vi "GageLv_Core.vi"(8 "error in":errorcluster, 9 "SignalBuffer queue in":refnum<queue>, 10 "Gage CtrlQueue in":refnum<queue>) -> (0 "error out":errorcluster)   [LabVIEW 2014, in "GageLv.lvlib"]
uses:
  <instrlib>/GageLv_uic/GageLv.lvlib
  <instrlib>/GenericDAQ/VI/GenericDAQ_Ctrl_Queue.ctl
  <instrlib>/GenericDAQ/VI/GenericDAQ_State.ctl
  <instrlib>/GenericDAQ/VI/GenericDAQ_Signal.ctl
  <instrlib>/GageLv_uic/VI/Gage_Configs.ctl
  <instrlib>/GageLv_uic/VI/Gage_PrivateStats.ctl
  <instrlib>/GageLv_uic/VI/Gage_DAQStatus.ctl
  <vilib>/Utility/error.llb/DialogType.ctl
  <instrlib>/GageLv_uic/VI/SetSecondaryDataVIRef_Typedef.ctl
  <vilib>/Utility/error.llb/Error Cluster From Error Code.vi
  <vilib>/ErrorRing/Error Ring.xnode
  <userlib>/Utility/ErrorLog_lib.lvlib
  <instrlib>/GenericDAQ/GenericDAQ.lvlib
panel:
  in  "StartAll":bool
  out "Core#":i32
  in  "Get_ConfigAll":bool
  out "LiveStat":T1
  in  "Gage_Config":T3={"Acquisition"={"Sample Rate"=1000000000.0, "Mode"=0, "Start (0)"=0.0, "Depth"=32768.0, "Segment Size"=32768.0, "Trigger Delay"=0.0, "Trigger Timeout"=-1.0, "Trigger Holdoff"=0.0, "Clock mode"=enum."Internal", "Segment"=1}, "Channels"=[{"Coupling"=1, "Differential Input"=FALSE, "Direct-to-ADC"=FALSE, "Range"=2000, "Impedance"=50, "DC Offset"=0, "Filter"=0}], "Trigger"={"Slope"=0, "Level"=25, "Source"=0, "External Range"=2000, "External Coupling"=0, "External"=TRUE, "Disable"=FALSE, "External Impedance"=0}, "Mode(Gage)"=enum."Continuous"} {"Trigger"."External Impedance" items=["50 Ohm", "HiZ"]; "Trigger"."External Coupling" items=["DC", "AC"]; "Trigger"."External Range" min=2000 max=10000 step=8000; "Trigger"."Slope" items=["Rising", "Falling"]; "Trigger"."Level" min=-100 max=100; "Trigger"."Source" min=0 max=64 step=1; "Channels"."Impedance" min=50 max=1000000 step=999950; "Channels"."Coupling" items=["DC", "AC"]; "Acquisition"."Start (0)" min=-1000000.0 max=0.0 step=16.0; "Acquisition"."Segment Size" min=256.0 step=128.0; "Acquisition"."Trigger Delay" min=0.0 step=128.0; "Acquisition"."Trigger Timeout" format="%.0p"; "Acquisition"."Trigger Holdoff" min=0.0 step=128.0; "Acquisition"."Depth" min=256.0 step=128.0; "Acquisition"."Mode" items=["Single", "Dual", "Quad", "Octal"]; "Acquisition"."Sample Rate" format="%.0p"}
  out "Graph":sgl[](graph)
  in  "fConfig":bool
  in  "Reset":bool
  in  "CloseAll":bool
  in  "Close":bool
  in  "Enumerate":bool
  in  "Open":bool
  in  "Quit":bool
  in  "Start":bool
  in  "ConfigAll":bool
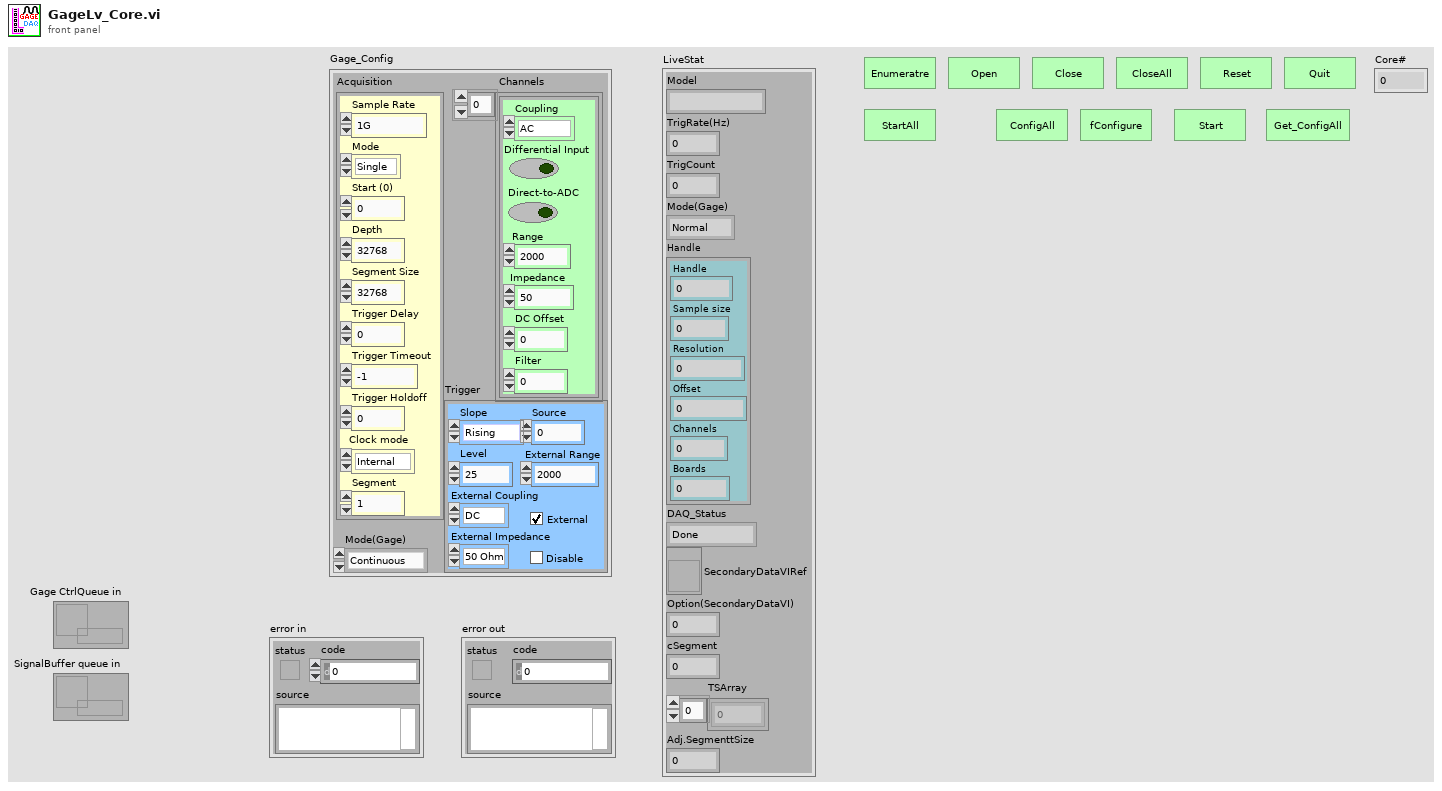
[diagram p1: front panel]
types:
  T1 = typedef "GageLv.lvlib/Gage_PrivateStats.ctl" = cluster{"Model":string, "TrigRate(Hz)":dbl, "TrigCount":i32, "Mode(Gage)":enum16{"Normal", "Continuous", "MultiRecord", "HwAverage"}, "Handle":cluster{"Handle":u32, "Sample size":u32, "Resolution":i32, "Offset":i32, "Channels":u32, "Boards":u32}, "DAQ_Status":T2, "SecondaryDataVIRef":refnum<vi>, "Option(SecondaryDataVI)":i32, "cSegment":i32, "TSArray":dbl[], "Adj.SegmenttSize":dbl}
  T2 = typedef "GageLv.lvlib/Gage_DAQStatus.ctl" = enum16{"Done", "Armed", "Triggered", "Transfering"}
  T3 = typedef "GageLv.lvlib/Gage_Configs.ctl" = cluster{"Acquisition":cluster{"Sample Rate":dbl, "Mode":u16, "Start (0)":dbl, "Depth":dbl, "Segment Size":dbl, "Trigger Delay":dbl, "Trigger Timeout":dbl, "Trigger Holdoff":dbl, "Clock mode":enum16{"Internal", "External", "Reference"}, "Segment":u32}, "Channels":cluster{"Coupling":u16, "Differential Input":bool, "Direct-to-ADC":bool, "Range":u32, "Impedance":u32, "DC Offset":i32, "Filter":i32}[], "Trigger":cluster{"Slope":u16, "Level":i32, "Source":i32, "External Range":u32, "External Coupling":u16, "External":bool, "Disable":bool, "External Impedance":u16}, "Mode(Gage)":enum16{"Normal", "Continuous", "MultiRecord", "HwAverage"}}
  T4 = enum16{"Normal", "MultiRecStart", "MultiRecEnd", "Reserved1", "Reserved2", "Reserved3"}
  T5 = typedef "DialogType.ctl" = u16
  T6 = typedef "GenericDAQ.lvlib/GenericDAQ_Signal.ctl" = cluster{"tickcount":u32, "Signal":sgl[], "SecondaryData":dbl[], "Flag":enum16{"Normal", "LineStart", "LineEnd", "FrameStart", "FrameEnd", "Reserved1", "Reserved2"}, "Segment#":i32}
  T7 = enum16{"Normal", "Continuous", "MultiRecord", "HwAverage"}
  T8 = typedef "GenericDAQ.lvlib/GenericDAQ_Ctrl_Queue.ctl" = cluster{"GenericDAQ State":T9, "Variant":variant}
  T9 = typedef "GenericDAQ.lvlib/GenericDAQ_State.ctl" = enum16{"Enumerate", "Open", "Close", "CloseAll", "Reset", "Quit", "==Settings==", "SetAcquisition_", "SetChannels_", "SetTrigger_", "SetAnalogTrigDetector_", "SetAll_AcquChTrig_", "fConfigurate", "fStart", "GetStatus", "_WaitForDone/Idle", "_GetData", "GetAcquisition", "GetChannels", "GetTrigger", "GetAll_AcquChTrig", "Abort", "==Messaging==", "_PushDataOut", "GetStat_", "GetConfig_", "==ModeSetup==", "SetSignalBuffer_", "SetMode_", "SetSecondaryDataRef._", "SetDynamicBuffer_", "==AnalogOut==", "GetChannelCount_AO", "fStart_AO", "SetChEnable_AO", "SetConfig_AO", "SetFuncData_AO", "SetOffset_AO_", "SetMasterNode_AO", "SetStates_AO", "SetSymetry_AO", "SetTriggerSource_AO", "==Trigger==", "ManualTrigger", "===Sync===", "LineStart", "LineEnd", "FrameStart", "FrameEnd", "EOL_PassThrough", "SOL_PassThrough"}
  T10 = typedef "SetSecondaryDataVIRef_Typedef.ctl" = cluster{"SecondaryDataVIRef.":refnum<vi>, "Option":i32}
  T11 = cluster{"Handle":u32, "Sample size":u32, "Resolution":i32, "Offset":i32, "Channels":u32, "Boards":u32}
  T12 = cluster{"Sample Rate":dbl, "Mode":u16, "Start (0)":dbl, "Depth":dbl, "Segment Size":dbl, "Trigger Delay":dbl, "Trigger Timeout":dbl, "Trigger Holdoff":dbl, "Clock mode":enum16{"Internal", "External", "Reference"}, "Segment":u32}
  T13 = cluster{"Sample Rate":dbl, "Clock mode":enum16{"Internal", "External", "Reference"}, string, "Depth":dbl, "Segment Size":dbl, "Trigger Timeout":dbl, "Trigger Holdoff":dbl, "Trigger Delay":dbl}
  T14 = cluster{"Coupling":u16, "Differential Input":bool, "Direct-to-ADC":bool, "Range":u32, "Impedance":u32, "DC Offset":i32, "Filter":i32}[]
  T15 = cluster{string, "Differential Input":bool, "Direct-to-ADC":bool, "Range":u32, "Impedance":u32, "DC Offset":i32, "Filter":i32}
  T16 = cluster{"Slope":u16, "Level":i32, "Source":i32, "External Range":u32, "External Coupling":u16, "External":bool, "Disable":bool, "External Impedance":u16}
  T17 = cluster{string, "Level":i32, "Source":i32, "External Range":u32, string, "External":bool, "Disable":bool, string}
  T18 = cluster{string, "Level":i32, "Source":i32, "External Range":u32, string, "External":bool, "Disable":bool, string}[]
  T19 = cluster{"Handle":u32, "Sample Size":u32, "Resolution":i32, "Offset":i32, "Channels":u32, "Boards":u32}
  T20 = cluster{"Coupling":u16, "Differential Input":bool, "Direct-to-ADC":bool, "Range":u32, "Impedance":u32, "DC Offset":i32, "Filter":i32}
  T21 = typedef "Gage.lvlib/Gage_Configs.ctl" = cluster{"Acquisition":cluster{"Sample Rate":dbl, "Mode":u16, "Start (0)":dbl, "Depth":dbl, "Segment Size":dbl, "Trigger Delay":dbl, "Trigger Timeout":dbl, "Trigger Holdoff":dbl, "Clock mode":enum16{"Internal", "External", "Reference"}, "Segment":u32}, "Channels":cluster{"Coupling":u16, "Differential Input":bool, "Direct-to-ADC":bool, "Range":u32, "Impedance":u32, "DC Offset":i32, "Filter":i32}[], "Trigger":cluster{"Slope":u16, "Level":i32, "Source":i32, "External Range":u32, "External Coupling":u16, "External":bool, "Disable":bool, "External Impedance":u16}, "Mode(Gage)":enum16{"Normal", "Continuous", "MultiRecord", "HwAverage"}}
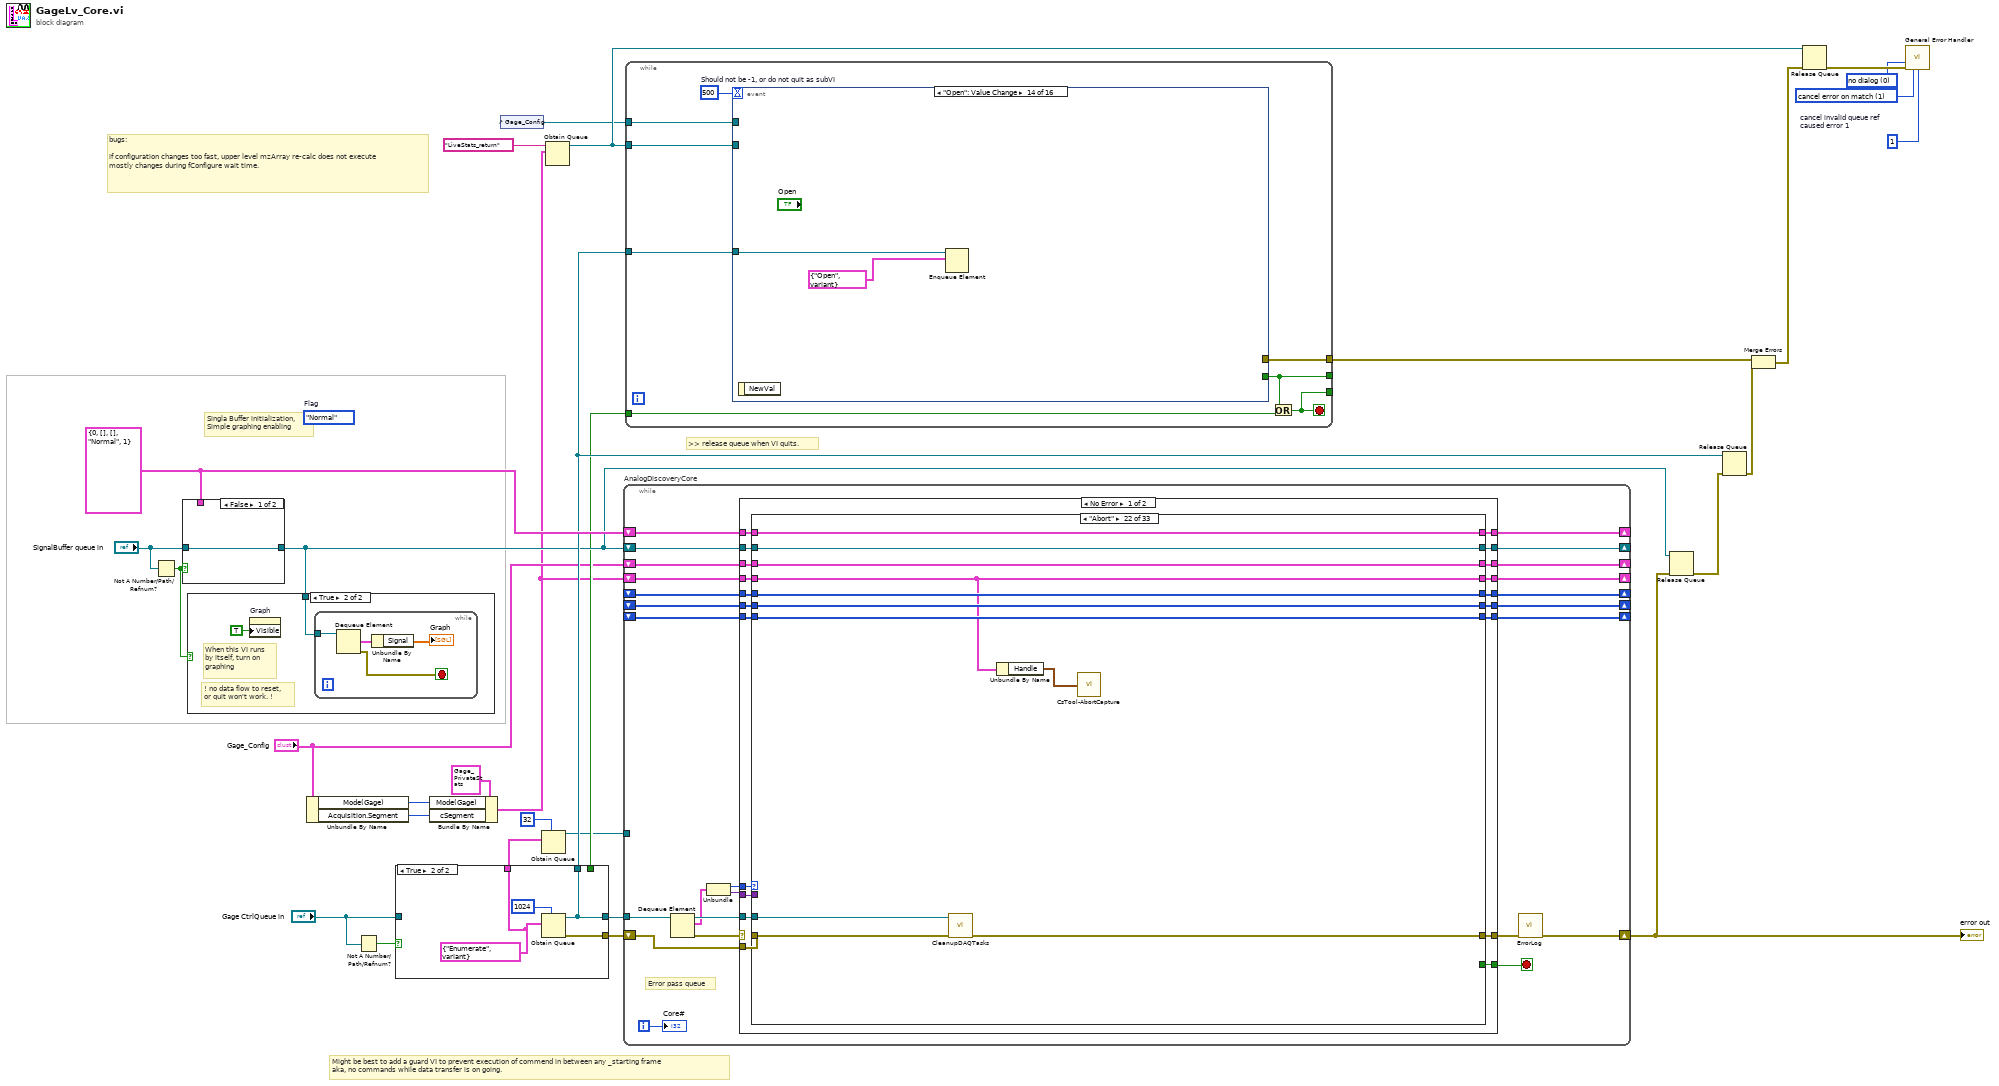
[diagram p0: block diagram]
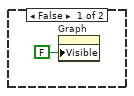
[diagram p2: hidden frame]
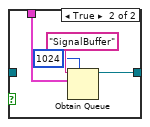
[diagram p3: hidden frame]
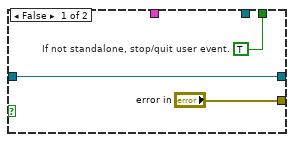
[diagram p4: hidden frame]
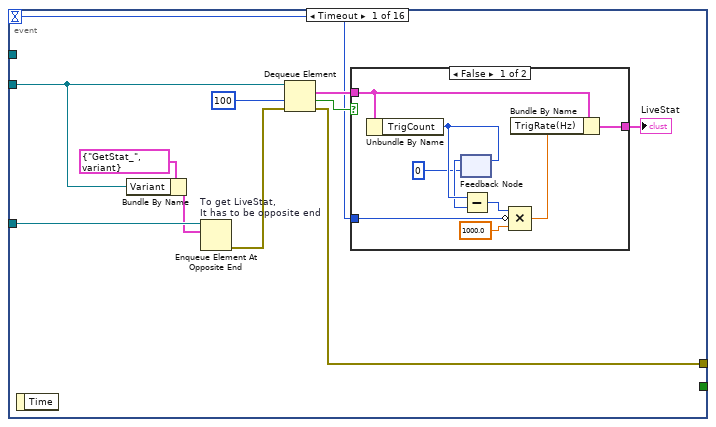
[diagram p5: hidden frame]
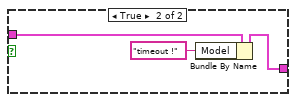
[diagram p6: hidden frame]
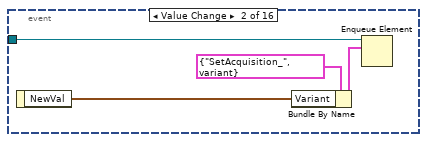
[diagram p7: hidden frame]
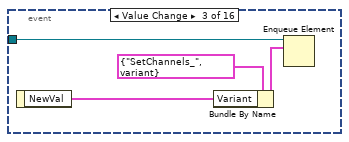
[diagram p8: hidden frame]
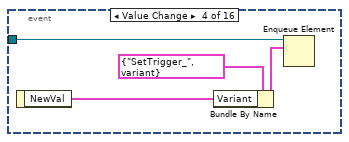
[diagram p9: hidden frame]
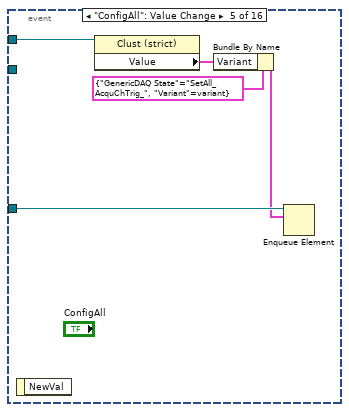
[diagram p10: hidden frame]
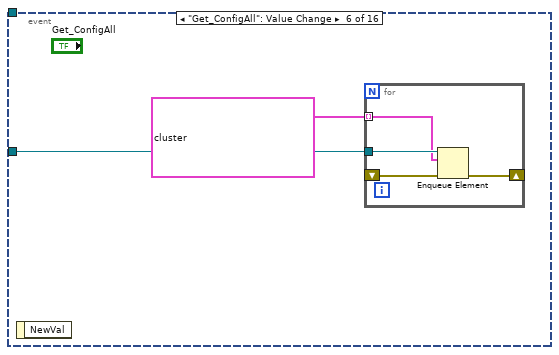
[diagram p11: hidden frame]
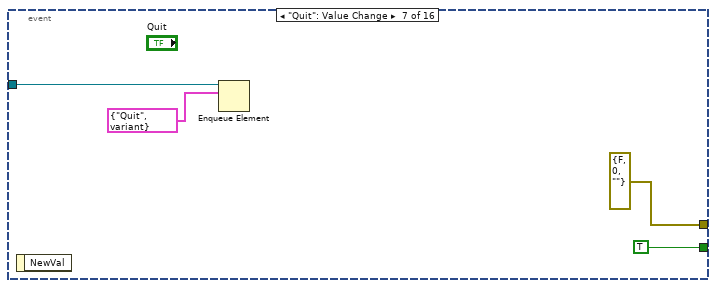
[diagram p12: hidden frame]
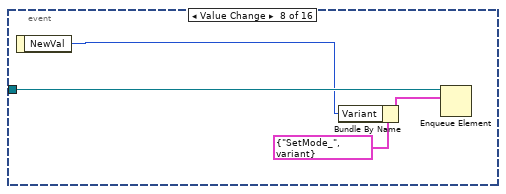
[diagram p13: hidden frame]
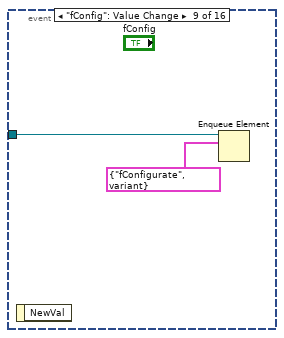
[diagram p14: hidden frame]
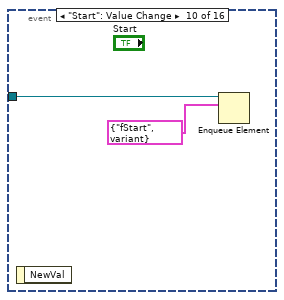
[diagram p15: hidden frame]
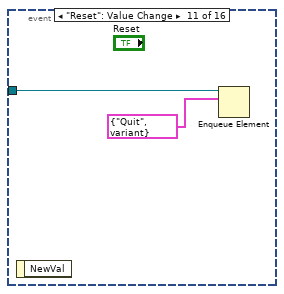
[diagram p16: hidden frame]
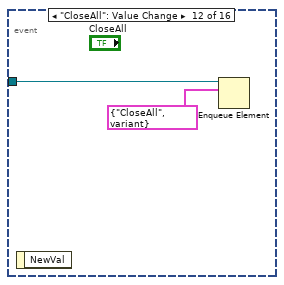
[diagram p17: hidden frame]
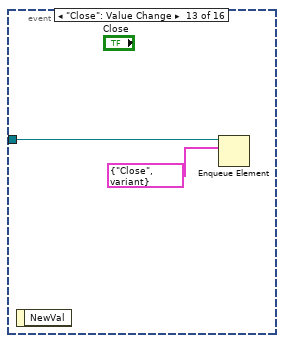
[diagram p18: hidden frame]
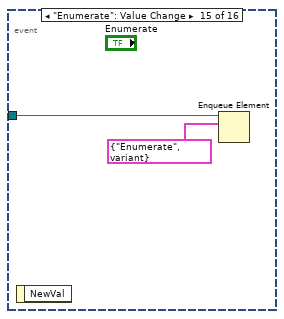
[diagram p19: hidden frame]
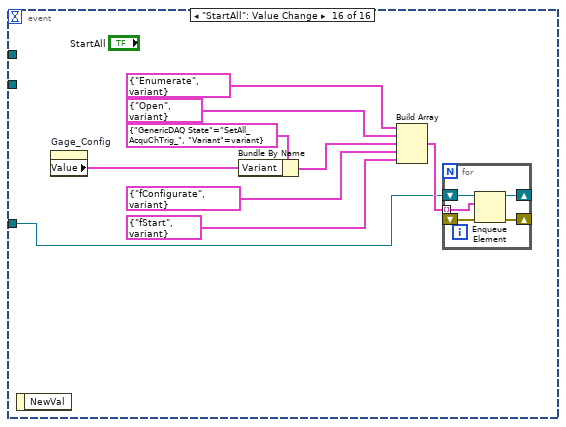
[diagram p20: hidden frame]
diagram:
  (unwired) T4."Normal"  # Flag
  w12 = 1  # cancel invalid queue ref caused error 1
  w13 = 1 items=["no exception", "cancel error on match", "set error on match"] ("[exception action] (none:0)")
  w14 = T5 0 items=["no dialog", "OK message", "continue or stop message", "OK message + warnings", "continue/stop + warnings"] ("type of dialog (OK msg:1)")
  w30 = T6 {"tickcount"=0, "Signal"=[], "SecondaryData"=[], "Flag"=enum."Normal", "Segment#"=1} ("Signal_Typedef")
  # "Might be best to add a guard VI to prevent execution of commend in between any _starting frame \naka, no commands while data transfer is on going."
  # "bugs:\n\nif configuration changes too fast, upper level mzArray re-calc does not execute\nmostly changes during fConfigure wait time."
  # "Singla Buffer initialization,\nSimple graphing enabling"
  # ">> release queue when VI quits."
  n1 = Not A Number/Path/Refnum?(number/path/refnum="SignalBuffer queue in") -> (NaN/Path/Refnum?=w17:bool)
  n2 = case shown="False" w17 {
    tunnel: w30 -> [_ w35]
    tunnel: [w31 w32] -> w18
    tunnel: "SignalBuffer queue in" -> [w31 _]
    frame False {
    }
    frame True {
      n3 = Obtain Queue(max queue size (-1, unlimited)=1024, name (unnamed)="SignalBuffer", element data type=w35) -> (queue out=w32:refnum<queue>)  [unwired: 2 in, 2 out]
    }
  }
  n4 = case shown="True" w17 {
    tunnel: w18 -> [_ w38]
    frame False {
      n5 = property on="Graph" class="WFGraph (strict)"("Visible"=FALSE) -> ()  [unwired: 2 in, 2 out]
    }
    frame True {
      # "! no data flow to reset,\nor quit won't work. !"
      # "When this VI runs\nby itself, turn on \ngraphing"
      n6 = property on="Graph" class="WFGraph (strict)"("Visible"=TRUE) -> ()  [unwired: 2 in, 2 out]
      n7 = while {
        tunnel: w38 -> [w42]
        stop <- w39 stop-if-true
        n8 = Dequeue Element(queue=w42) -> (element=w41:T6, error out=w39:errorcluster)  [unwired: 2 in, 2 out]
        n9 = Unbundle By Name(w41) -> ("Signal"=→"Graph":sgl[])
      }
    }
  }
  n10 = Unbundle By Name("Gage_Config") -> ("Mode(Gage)"=w8:T7, "Acquisition.Segment"=w1:u32)
  n11 = Not A Number/Path/Refnum?(number/path/refnum="Gage CtrlQueue in") -> (NaN/Path/Refnum?=w27:bool)
  n12 = case shown="True" w27 {
    tunnel: [w45 w47] -> w29
    tunnel: ["error in" w49] -> w28
    tunnel: "Gage CtrlQueue in" -> [w45 _]
    tunnel: [_ w47] -> w23
    tunnel: [w43 _] -> w11
    tunnel: [_ w46] -> w4
    frame False {
      w43 = TRUE  # If not standalone, stop/quit user event.
    }
    frame True {
      w46 = T8 {"GenericDAQ State"=enum."Enumerate", "Variant"=variant}
      n13 = Obtain Queue(max queue size (-1, unlimited)=1024, element data type=w46) -> (queue out=w47:refnum<queue>, error out=w49:errorcluster)  [unwired: 3 in, 1 out]
    }
  }
  n14 = Bundle By Name(cluster=T1 {"Model"="", "TrigRate(Hz)"=0.0, "TrigCount"=0, "Mode(Gage)"=enum."Normal", "Handle"={"Handle"=0, "Sample size"=0, "Resolution"=0, "Offset"=0, "Channels"=0, "Boards"=0}, "DAQ_Status"=enum."Done", "SecondaryDataVIRef"=refnum, "Option(SecondaryDataVI)"=0, "cSegment"=0, "TSArray"=[], "Adj.SegmenttSize"=0.0} ("PrivateStats(Live)"), "Mode(Gage)"=w8, "cSegment"=w1) -> (w5:T1)
  n15 = control-ref of="Gage_Config"() -> (w6:refnum<vi>)
  n16 = Obtain Queue(max queue size (-1, unlimited)=32, element data type=w4) -> (queue out=w3:refnum<queue>)  [unwired: 3 in, 2 out]
  n17 = Obtain Queue(name (unnamed)="LiveStats_return", element data type=w5) -> (queue out=w21:refnum<queue>)  [unwired: 3 in, 2 out]
  n18 = while "AnalogDiscoveryCore" {
    shift-right: [w73] -> _
    shift-left: w18 -> [w74]
    tunnel: w29 -> [w60]
    shift-right: [w50] -> w16
    shift-left: w28 -> [w62]
    shift-right: [w71] -> _
    shift-left: "Gage_Config" -> [w70]
    shift-right: [w54] -> _
    shift-left: w5 -> [w69]
    shift-right: [w63] -> _
    shift-left: _ -> [w67]
    shift-right: [w64] -> _
    shift-left: w30 -> [w68]
    shift-right: [w57] -> _
    shift-left: _ -> [w55]
    shift-right: [w58] -> _
    shift-left: _ -> [w56]
    tunnel: w3 -> [_]
    i -> [w52]
    stop <- w72 stop-if-true
    # "Error pass queue"
    n19 = Dequeue Element(queue=w60) -> (queue out=w59:refnum<queue>, element=w53:T8, error out=w61:errorcluster)  [unwired: 2 in, 1 out]
    n20 = Unbundle(w53) -> ("GenericDAQ State"=w66:T9, "Variant"=w65:variant)
    n21 = case shown="No Error" w61 {
      tunnel: w74 -> [w94 w1020]
      tunnel: [w93 w1020] -> w73
      tunnel: [w92 TRUE] -> w72
      tunnel: [w91 w1018] -> w51
      tunnel: [w90 w1021] -> w71
      tunnel: w70 -> [w89 w1021]
      tunnel: w69 -> [w88 w1022]
      tunnel: w68 -> [w87 w1019]
      tunnel: w67 -> [w86 w1023]
      tunnel: w59 -> [w85 _]
      tunnel: w66 -> [w84 _]
      tunnel: w65 -> [w83 _]
      tunnel: [w82 w1019] -> w64
      tunnel: [w81 w1023] -> w63
      tunnel: [w80 w1022] -> w54
      tunnel: w62 -> [w79 _]
      tunnel: [w78 w1017] -> w58
      tunnel: [w77 w1016] -> w57
      tunnel: w56 -> [w76 w1017]
      tunnel: w55 -> [w75 w1016]
      frame No Error {
        n22 = case shown="\"Abort\"" w84 {
          tunnel: w94 -> [w102 w111 w140 w153 w169 w184 w201 w219 w242 w313 w368 w423 w468 w491 w507 w529 w585 w675 w690 w733 w744 w759 w767 w800 w887 w900 w913 w926 w952 w966 w997 w998 w1007]
          tunnel: [w102 w111 w140 w153 w169 w184 w201 w219 w242 w313 w368 w423 w468 w491 w507 w529 w585 w675 w690 w733 w744 w759 w767 w800 w887 w900 w913 w927 w952 w966 w997 w998 w1007] -> w93
          tunnel: [_ _ _ _ _ _ w195 _ _ _ _ _ _ _ _ _ _ _ _ _ _ _ _ _ _ _ _ _ _ _ _ _ _] -> w92
          tunnel: w85 -> [_ _ _ _ _ w180 w192 _ w225 w299 w354 w420 w455 w485 _ w531 w581 _ _ _ w737 w751 _ w796 _ _ _ _ _ _ _ _ _]
          tunnel: w79 -> [w101 w107 w136 w147 w168 w179 w193 _ w234 w304 w359 w414 w456 w475 w503 w530 w579 w674 w689 w732 w736 w750 _ w798 w881 w891 _ w923 w942 _ w996 w1006 w1015]
          tunnel: [w101 w107 errorcluster {"status"=FALSE, "code"=0, "source"=""} ("error out") w142 w161 w178 w194 w214 w230 w305 w360 w419 w453 w479 w503 w524 w582 w652 w678 w707 w735 w749 w762 w797 w880 w892 w908 w924 w943 w954 w996 w1006 w1015] -> w91
          tunnel: [w100 w110 w139 w152 w167 w183 w200 w218 w239 w310 w365 w417 w467 w490 w506 w528 w587 w669 w685 w725 w740 w758 w766 w791 w879 w893 w912 w932 w951 w965 w995 w1005 w1014] -> w90
          tunnel: w89 -> [w100 w110 w139 w152 w167 w183 w200 w218 w237 w308 w363 w417 w467 w490 w506 w528 w587 w671 w683 w731 w740 w758 w766 w791 w879 w893 w912 w932 w951 w965 w995 w1005 w1014]
          tunnel: [w99 w109 w131 w149 w162 w177 w197 w217 w240 w311 w366 w411 w465 w488 w502 w521 w554 w665 w684 w726 w743 w752 w765 w781 w876 w899 w911 w931 w948 w960 w994 w1004 w1013] -> w80
          tunnel: w88 -> [w99 w109 w137 w150 w162 w177 w197 w217 w240 w311 w366 w411 w465 w488 w498 w522 w576 w670 w684 w726 w743 w752 w765 w782 w876 w899 w911 w931 w947 w955 w994 w1004 w1013]
          tunnel: w87 -> [w98 w108 w138 w151 w166 w182 w199 w216 w241 w312 w367 w422 w466 w489 w505 w527 w584 w673 w688 w730 w742 w757 w764 w775 w886 w898 w910 w930 w950 w964 w993 w1003 w1012]
          tunnel: w86 -> [w97 w106 _ w148 w165 w181 w198 w215 w231 w302 w357 w421 w464 w484 w504 w523 w586 w672 w687 w729 w741 w756 w763 w789 w885 w897 w909 w929 w949 w963 w992 w1002 w1011]
          tunnel: w83 -> [_ _ w135 _ _ _ _ _ w238 w309 w364 w418 _ _ _ _ _ _ _ _ _ _ _ _ w882 w896 _ w928 w946 w958 _ _ _]
          tunnel: [w98 w108 w138 w151 w166 w182 w199 w216 w241 w312 w367 w422 w466 w489 w505 w527 w583 w673 w688 w730 w742 w757 w764 w775 w886 w898 w910 w930 w950 w964 w993 w1003 w1012] -> w82
          tunnel: [w97 w106 w115 w148 w165 w181 w198 w215 w232 w302 w357 w421 w464 w484 w504 w523 w578 w672 w687 w729 w741 w756 w763 w788 w885 w897 w909 w929 w949 w963 w992 w1002 w1011] -> w81
          tunnel: [w96 w104 w114 w146 w164 w171 w191 w213 w229 w301 w356 w413 w462 w483 w501 w511 w570 w659 w680 w728 w739 w755 w761 w786 w878 w890 w907 w920 w941 w962 w991 w1001 w1010] -> w78
          tunnel: [w95 w103 w113 w145 w163 w170 w190 w212 w228 w300 w355 w412 w461 w482 w500 w510 w569 w658 w679 w727 w738 w754 w760 w784 w877 w889 w906 w919 w940 w961 w990 w1000 w1009] -> w77
          tunnel: w76 -> [w96 w104 _ w146 w164 w171 w191 w213 w227 w301 w356 w413 w462 w483 w501 w511 w573 w659 w680 w728 w739 w755 w761 w787 w878 w890 w907 w920 w941 w962 w991 w1001 w1010]
          tunnel: w75 -> [w95 w103 _ w145 w163 w170 w190 w212 w226 w300 w355 w412 w461 w482 w500 w510 w572 w658 w679 w727 w738 w754 w760 w785 w877 w889 w906 w919 w940 w961 w990 w1000 w1009]
          frame Default {
          }
          frame "Enumerate" {
            n23 = call <instrlib>:"CsTool-Initialize.vi"() -> ("Number Of Systems"=w105:i32)  [unwired: 1 out]
            n24 = call <instrlib>:"CsTool-ErrorHandler.vi"("Error Code"=w105) -> ()  [unwired: 2 in, 1 out]
          }
          frame "Open" {
            n25 = Variant To Data(error in=w136, type="", Variant=w135) -> (data=w130:string, error out=w133:errorcluster)
            n26 = Select(t="any", s=TRUE, f=w130) -> (s? t:f=w129:string)
            n27 = call <instrlib>:"CsTool-GetSystem.vi"("Board Name (Any)"=w129) -> ("Error Code"=w132:i32, "Handle Cluster"=w121:T11)  [unwired: 3 in]
            n28 = call <instrlib>:"CsTool-GetSystemName.vi"("Handle Cluster"=w121) -> ()  [unwired: 2 out]
            n29 = call <instrlib>:"CsTool-ErrorHandler.vi"("Error Code"=w132, "Handle Cluster"=w121) -> ("Error String"=w122:string)  [unwired: 1 in]
            n30 = call <instrlib>:"CsTool-GetSystemInfo.vi"("Handle Cluster"=w121) -> ()  [unwired: 7 out]
            n31 = Bundle By Name(cluster=w137, "Handle"=w121, "Model"=w129, "TrigRate(Hz)"=0.0, "TrigCount"=0) -> (w131:T1)
            n32 = Bundle By Name(cluster=w133, "source"=w122) -> ()  [unwired: 1 out]
            n33 = Wait (ms)(milliseconds to wait=u32 0) -> ()  [unwired: 1 out]
            n34 = Multiply(x=2 ("16KSa, per spec"), y=262144 ("dimension size")) -> (x*y=w116:i32)
            n35 = Initialize Array(0 ("Numeric"), w116) -> (w115:i32[])
            n36 = Initialize Array(i16 0 ("Numeric"), w116) -> (w114:i16[])
            n37 = Initialize Array(u8 0 ("Numeric"), w116) -> (w113:u8[])
          }
          frame "Close" {
            n38 = Unbundle By Name(w150) -> ("Handle"=w143:T11)
            n39 = call <instrlib>:"CsTool-AbortCapture.vi"("Handle Cluster"=w143) -> ("Error Code"=w144:i32)
            n40 = call <instrlib>:"CsTool-ErrorHandler.vi"("Error Code"=w144, "Handle Cluster"=w143) -> ("Error String"=w141:string)  [unwired: 1 in]
            n41 = disable-structure shown="Enabled" {
              disable-tunnel: w150 -> [w156 w157]
              disable-tunnel: [w155 w157] -> w149
              frame Enabled {
                n42 = Bundle By Name(cluster=w156, "Handle.Handle"=u32 0) -> (w155:T1)
              }
              frame Disabled {
              }
            }
            n43 = Bundle By Name(cluster=w147, "source"=w141) -> (w142:errorcluster)
          }
          frame "CloseAll" {
            # "not really useful here."
            n44 = Unbundle By Name(w162) -> ("Handle"=w160:T11)
            n45 = call <instrlib>:"CsTool-AbortCapture.vi"("Handle Cluster"=w160) -> ("Error Code"=w159:i32)
            n46 = call <instrlib>:"CsTool-ErrorHandler.vi"("Error Code"=w159, "Handle Cluster"=w160) -> ("Error String"=w158:string)  [unwired: 1 in]
            n47 = Bundle By Name(cluster=w168, "source"=w158) -> (w161:errorcluster)
          }
          frame "Reset" {
            n48 = Unbundle By Name(w177) -> ("Model"=w175:string)
            n49 = Bundle By Name(cluster=T8 {"GenericDAQ State"=enum."Open", "Variant"=variant} ("element"), "Variant"=w175) -> (w174:T8)
            n50 = Build Array(w174, T8 {"GenericDAQ State"=enum."Close", "Variant"=variant} ("element")) -> (w172:T8[])
            n51 = for {
              tunnel: w180 -> [w188]
              tunnel: w172 -> [w185] mode=indexing
              shift-right: [w186] -> w178
              shift-left: w179 -> [w187]
              n52 = Enqueue Element At Opposite End(queue=w188, element=w185, error in (no error)=w187) -> (error out=w186:errorcluster)  [unwired: 1 in, 2 out]
            }
          }
          frame "Quit" {
            n53 = Unbundle By Name(w197) -> ("Handle"=w189:T11, "Handle.Handle"=w196:u32)
            n54 = case "Check handle leak??" shown="Default" w196 {
              tunnel: [_ TRUE] -> w195
              tunnel: [w203 _] -> w194
              tunnel: w193 -> [w204 _]
              tunnel: w192 -> [w205 _]
              tunnel: w189 -> [_ w210]
              frame Default {
                n55 = for {
                  tunnel: w205 -> [w209]
                  tunnel: T8[] [{"GenericDAQ State"=enum."Quit", "Variant"=variant}, {"GenericDAQ State"=enum."Close", "Variant"=variant}] -> [w206] mode=indexing
                  shift-right: [w207] -> w203
                  shift-left: w204 -> [w208]
                  n56 = Enqueue Element At Opposite End(queue=w209, element=w206, error in (no error)=w208) -> (error out=w207:errorcluster)  [unwired: 1 in, 2 out]
                }
              }
              frame 0 {
                n57 = call <instrlib>:"CsTool-FreeSystem.vi"("Handle Cluster"=w210) -> ()  [unwired: 1 out]
              }
            }
          }
          frame "==Settings==" {
            # "Invalid frame"
            n58 = xnode "Error Ring"() -> ("error out"=w214:errorcluster)
          }
          frame "SetAcquisition_" {
            n59 = Unbundle By Name(w237) -> ("Acquisition"=w236:T12)
            n60 = Variant To Data(error in=w234, type=w236, Variant=w238) -> (data=w235:T12, error out=w233:errorcluster)
            n61 = Bundle By Name(cluster=w237, "Acquisition"=w235) -> (w239:T3)
            n62 = case shown="No Error" w233 {
              selector: w233 -> [w250 _]
              tunnel: w240 -> [w277 _]
              tunnel: w235 -> [w270 _]
              tunnel: [w263 w293] -> w232
              tunnel: w231 -> [_ w293]
              tunnel: [w260 w292] -> w230
              tunnel: [w262 w291] -> w229
              tunnel: [w261 w290] -> w228
              tunnel: w227 -> [_ w291]
              tunnel: w226 -> [_ w290]
              tunnel: w225 -> [w251 _]
              frame No Error {
                n63 = call <instrlib>:"CleanupDAQTasks.vi"("error in (no error)"=w250, "Queue in"=w251) -> ("error out"=w249:errorcluster)  [unwired: 8 in, 1 out]
                n64 = Unbundle By Name(w270) -> ("Segment"=w246:u32, "Mode"=w257:u16, "Sample Rate"=w276:dbl, "Clock mode"=w275:enum16{"Internal", "External", "Reference"})
                n65 = Unbundle By Name(w270) -> ("Depth"=w267:dbl, "Segment Size"=w274:dbl, "Trigger Timeout"=w273:dbl, "Trigger Holdoff"=w272:dbl, "Trigger Delay"=w271:dbl)
                n66 = Unbundle By Name(w277) -> ("Handle"=w259:T11)
                n67 = flat-sequence {
                  tunnel: w259 -> [w281]
                  tunnel: [w281] -> _
                  tunnel: [w281] -> w247
                  tunnel: [w282] -> w248
                  tunnel: w247 -> [w282]
                  tunnel: w248 -> [w289]
                  tunnel: w246 -> [w288]
                  tunnel: w245 -> [w287]
                  tunnel: [w286] -> w244
                  tunnel: [w285] -> w243
                  frame #0 {
                    n68 = call <instrlib>:"CsTool-AbortCapture.vi"("Handle Cluster"=w281) -> ()  [unwired: 1 out]
                  }
                  frame #1 {
                    n69 = Wait (ms)(milliseconds to wait=u32 5) -> ()  [unwired: 1 out]
                  }
                  frame #2 {
                    n70 = call <instrlib>:"CsTool-ConfigureAcquisition.vi"("Handle Cluster"=w289, "Segment Count (1)"=w288, "Acquisition"=w287) -> ("Error Code"=w285:i32)  [unwired: 2 in]
                    n71 = call <instrlib>:"CsTool-ErrorHandler.vi"("StopOnError (true)"=FALSE, "Error Code"=w285, "Handle Cluster"=w289) -> ("Error String"=w286:string)
                  }
                }
                n72 = Index Array(array=string[] ["Single", "Dual", "Quad", "Octal"], index=w257) -> (element=w268:string)
                n73 = Scale By Power Of 2(n=w257, x=ext 1.0) -> (x*2^n=w258:ext)
                n74 = To Long Integer(number=w258) -> (32bit integer=w253:i32)
                n75 = Bundle("Sample Rate"=w276, "Clock mode"=w275, w268, "Depth"=w267, "Segment Size"=w274, "Trigger Timeout"=w273, "Trigger Holdoff"=w272, "Trigger Delay"=w271) -> (w245:T13)  [unwired: 1 in]
                n76 = Less Than 0?(x=w243) -> (x < 0?=w255:bool)
                n77 = To Long Integer(number=w267) -> (32bit integer=w266:i32)
                n78 = In Range and Coerce(upper limit=512000, x=w266, lower limit=1) -> (coerced(x)=w254:i32)  [unwired: 1 out]
                n79 = Multiply(x=w253, y=w254) -> (x*y=w252:i32)
                n80 = Initialize Array(0 ("Numeric"), w252) -> (w263:i32[])
                n81 = Initialize Array(i16 0 ("Numeric"), w252) -> (w262:i16[])
                n82 = Initialize Array(u8 0 ("Numeric"), w252) -> (w261:u8[])
                n83 = Bundle By Name(cluster=w249, "status"=w255, "source"=w244) -> (w260:errorcluster)
              }
              frame Error {
                n84 = xnode "Error Ring"() -> ("error out"=w292:errorcluster)
              }
            }
          }
          frame "SetChannels_" {
            n85 = Unbundle By Name(w308) -> ("Channels"=w307:T14)
            n86 = Variant To Data(error in=w304, type=w307, Variant=w309) -> (data=w306:T14, error out=w303:errorcluster)
            n87 = Bundle By Name(cluster=w308, "Channels"=w306) -> (w310:T3)
            n88 = case shown="No Error" w303 {
              selector: w303 -> [w324 _]
              tunnel: w311 -> [w327 _]
              tunnel: w306 -> [w326 _]
              tunnel: [w323 w348] -> w305
              tunnel: w299 -> [w320 _]
              frame No Error {
                n89 = call <instrlib>:"CleanupDAQTasks.vi"("error in (no error)"=w324, "Queue in"=w320) -> ("error out"=w321:errorcluster)  [unwired: 8 in, 1 out]
                n90 = for {
                  tunnel: w326 -> [w337] mode=indexing
                  shift-right: [w347] -> w325
                  shift-left: w321 -> [w347]
                  tunnel: [w336] -> w318 mode=indexing
                  n91 = Unbundle By Name(w337) -> ("Coupling"=w340:u16, "Differential Input"=w338:bool, "Direct-to-ADC"=w341:bool, "Range"=w342:u32, "Impedance"=w343:u32, "DC Offset"=w344:i32, "Filter"=w345:i32)
                  n92 = Index Array(array=string[] ["DC", "AC"] ("Strings []"), index=w340) -> (element=w339:string)
                  n93 = Bundle(w339, "Differential Input"=w338, "Direct-to-ADC"=w341, "Range"=w342, "Impedance"=w343, "DC Offset"=w344, "Filter"=w345) -> (w336:T15)  [unwired: 1 in]
                }
                n94 = Unbundle By Name(w327) -> ("Handle"=w322:T11)
                n95 = flat-sequence {
                  tunnel: w322 -> [w328]
                  tunnel: [w328] -> w317
                  tunnel: w317 -> [w330]
                  tunnel: [w330] -> w316
                  tunnel: w316 -> [w333]
                  tunnel: [w335] -> w319
                  tunnel: w318 -> [w334]
                  tunnel: [w331] -> w314
                  frame #0 {
                    n96 = call <instrlib>:"CsTool-AbortCapture.vi"("Handle Cluster"=w328) -> ()  [unwired: 1 out]
                  }
                  frame #1 {
                    n97 = Wait (ms)(milliseconds to wait=u32 5) -> ()  [unwired: 1 out]
                  }
                  frame #2 {
                    n98 = call <instrlib>:"CsTool-ConfigureChannelArray.vi"("Channels"=w334, "Handle Cluster"=w333) -> ("Error Code"=w331:u32)
                    n99 = call <instrlib>:"CsTool-ErrorHandler.vi"("StopOnError (true)"=FALSE, "Error Code"=w331, "Handle Cluster"=w333) -> ("Error String"=w335:string)
                  }
                }
                n100 = Less Than 0?(x=w314) -> (x < 0?=w315:bool)
                n101 = Bundle By Name(cluster=w325, "status"=w315, "source"=w319) -> (w323:errorcluster)
              }
              frame Error {
                n102 = xnode "Error Ring"() -> ("error out"=w348:errorcluster)
              }
            }
          }
          frame "SetTrigger_" {
            n103 = Unbundle By Name(w363) -> ("Trigger"=w362:T16)
            n104 = Variant To Data(error in=w359, type=w362, Variant=w364) -> (data=w361:T16, error out=w358:errorcluster)
            n105 = Bundle By Name(cluster=w363, "Trigger"=w361) -> (w365:T3)
            n106 = case shown="No Error" w358 {
              selector: w358 -> [w395 _]
              tunnel: w366 -> [w396 _]
              tunnel: w361 -> [w388 _]
              tunnel: [w378 w405] -> w360
              tunnel: w354 -> [w373 _]
              frame No Error {
                n107 = call <instrlib>:"CleanupDAQTasks.vi"("error in (no error)"=w395, "Queue in"=w373) -> ("error out"=w374:errorcluster)  [unwired: 8 in, 1 out]
                n108 = Unbundle By Name(w388) -> ("Slope"=w384:u16, "Level"=w391:i32, "Source"=w390:i32, "External Range"=w389:u32, "External Coupling"=w383:u16, "External"=w394:bool, "Disable"=w393:bool, "External Impedance"=w382:u16)
                n109 = Unbundle By Name(w396) -> ("Handle"=w377:T11)
                n110 = Index Array(array=string[] ["Rising", "Falling"] ("Strings [] 3"), index=w384) -> (element=w381:string)
                n111 = Index Array(array=string[] ["DC", "AC"] ("Strings [] 2"), index=w383) -> (element=w380:string)
                n112 = Index Array(array=string[] ["50 Ohm", "HiZ"] ("Strings []"), index=w382) -> (element=w379:string)
                n113 = flat-sequence {
                  tunnel: w377 -> [w397]
                  tunnel: [w397] -> w372
                  tunnel: w372 -> [w399]
                  tunnel: [w399] -> w371
                  tunnel: w371 -> [w402]
                  tunnel: w376 -> [w404]
                  tunnel: [w403] -> w375
                  tunnel: [w400] -> w369
                  frame #0 {
                    n114 = call <instrlib>:"CsTool-AbortCapture.vi"("Handle Cluster"=w397) -> ()  [unwired: 1 out]
                  }
                  frame #1 {
                    n115 = Wait (ms)(milliseconds to wait=u32 5) -> ()  [unwired: 1 out]
                  }
                  frame #2 {
                    n116 = call <instrlib>:"CsTool-ConfigureTriggerArray.vi"("Triggers"=w404, "Handle Cluster"=w402) -> ("Error Code"=w400:i32)
                    n117 = call <instrlib>:"CsTool-ErrorHandler.vi"("StopOnError (true)"=FALSE, "Error Code"=w400, "Handle Cluster"=w402) -> ("Error String"=w403:string)
                  }
                }
                n118 = Bundle(w381, "Level"=w391, "Source"=w390, "External Range"=w389, w380, "External"=w394, "Disable"=w393, w379) -> (w392:T17)  [unwired: 1 in]
                n119 = Build Array(w392) -> (w376:T18)
                n120 = Less Than 0?(x=w369) -> (x < 0?=w370:bool)
                n121 = Bundle By Name(cluster=w374, "status"=w370, "source"=w375) -> (w378:errorcluster)
              }
              frame Error {
                n122 = xnode "Error Ring"() -> ("error out"=w405:errorcluster)
              }
            }
          }
          frame "SetAll_AcquChTrig_" {
            n123 = Variant To Data(type=w417, Variant=w418) -> (data=w415:T3, error out=w416:errorcluster)  [unwired: 1 in]
            n124 = case shown="No Error" w416 {
              tunnel: w420 -> [w441 _]
              tunnel: [w440 w446] -> w419
              tunnel: w415 -> [w439 _]
              tunnel: w414 -> [w438 _]
              frame No Error {
                n125 = Unbundle By Name(w439) -> ("Mode(Gage)"=w428:T7, "Acquisition"=w436:T12, "Channels"=w434:T14, "Trigger"=w432:T16)
                n126 = Bundle By Name(cluster=T8 {"GenericDAQ State"=enum."SetMode_", "Variant"=variant} ("element"), "Variant"=w428) -> (w425:T8)
                n127 = Bundle By Name(cluster=T8 {"GenericDAQ State"=enum."SetAcquisition_", "Variant"=variant} ("element"), "Variant"=w436) -> (w426:T8)
                n128 = Bundle By Name(cluster=T8 {"GenericDAQ State"=enum."SetChannels_", "Variant"=variant} ("element"), "Variant"=w434) -> (w424:T8)
                n129 = Bundle By Name(cluster=T8 {"GenericDAQ State"=enum."SetTrigger_", "Variant"=variant} ("element"), "Variant"=w432) -> (w431:T8)
                n130 = Build Array(w425, w426, w424, w431) -> (w430:T8[])
                n131 = Reverse 1D Array(array=w430) -> (reversed array=w427:T8[])
                n132 = for "Has to be at the \nopposite end, otherwise\nrace condition" {
                  tunnel: w441 -> [w445]
                  shift-right: [w444] -> w440
                  shift-left: w438 -> [w443]
                  tunnel: w427 -> [w442] mode=indexing
                  n133 = Enqueue Element At Opposite End(queue=w445, element=w442, error in (no error)=w443) -> (error out=w444:errorcluster)  [unwired: 1 in, 2 out]
                }
              }
              frame Error {
                n134 = xnode "Error Ring"() -> ("error out"=w446:errorcluster)
              }
            }
          }
          frame "fConfigurate" {
            # "If dependancy of ErrorLog missing, \njust remove errorlog vi."
            # "fConfigurate => Commit (as in Gage SDK)"
            n135 = call <instrlib>:"CleanupDAQTasks.vi"("error in (no error)"=w456, "Queue in"=w455) -> ("error out"=w457:errorcluster)  [unwired: 8 in, 1 out]
            n136 = Unbundle By Name(w465) -> ("Handle"=w463:T11)
            n137 = flat-sequence {
              tunnel: w463 -> [w469]
              tunnel: [w469] -> w460
              tunnel: w460 -> [w472]
              tunnel: [w473] -> w458
              tunnel: [w471] -> w452
              frame #0 {
                n138 = disable-structure shown="Enabled" {
                  disable-tunnel: w469 -> [w470 _]
                  frame Enabled {
                    n139 = call <instrlib>:"CsTool-AbortCapture.vi"("Handle Cluster"=w470) -> ()  [unwired: 1 out]
                  }
                  frame Disabled {
                  }
                }
              }
              frame #1 {
                n140 = call <instrlib>:"CsTool-Commit.vi"("Handle Cluster"=w472) -> ("Error Code"=w471:i32)  [unwired: 2 in, 1 out]
                n141 = call <instrlib>:"CsTool-ErrorHandler.vi"("StopOnError (true)"=FALSE, "Error Code"=w471, "Handle Cluster"=w472) -> ("Error String"=w473:string)
              }
            }
            n142 = Less Than 0?(x=w452) -> (x < 0?=w454:bool)
            n143 = Bundle By Name(cluster=w457, "code"=w452, "status"=w454, "source"=w458) -> (w459:errorcluster)
            n144 = call <userlib>:"ErrorLog.vi"("error in (no error)"=w459) -> ("error out"=w453:errorcluster)  [unwired: 10 in]
          }
          frame "fStart" {
            # "Known issue:\n\nIf too manu fStart send here, virtual system crash.\nhas to restart Lv"
            # "Prevent program termination, \nwhen capture executed \nbefore previous one finished\n\nCould not find how to detect\na unfinished capture\n\nIn GetDate frame, capture actions is \nguarentted finished, no need to do so."
            n145 = call <instrlib>:"CleanupDAQTasks.vi"("error in (no error)"=w475, "Queue in"=w485) -> ("error out"=w476:errorcluster, "Queue out"=w477:refnum<queue>)  [unwired: 8 in]
            n146 = Unbundle By Name(w488) -> ("Handle"=w481:T11)
            n147 = flat-sequence {
              tunnel: w481 -> [w493]
              tunnel: [w493] -> w480
              tunnel: w480 -> [w495]
              tunnel: [w494] -> w478
              frame #0 {
                n148 = Wait (ms) "Prevent termination if too many \nfStart sent in short time."(milliseconds to wait=u32 50) -> ()  [unwired: 1 out]
                n149 = call <instrlib>:"CsTool-AbortCapture.vi"("Handle Cluster"=w493) -> ()  [unwired: 1 out]
              }
              frame #1 {
                n150 = call <instrlib>:"CsTool-Capture.vi"("Handle Cluster"=w495) -> ("Error Code"=w496:i32)
                n151 = call <instrlib>:"CsTool-ErrorHandler.vi"("Error Code"=w496, "Handle Cluster"=w495) -> ("Error String"=w494:string)  [unwired: 1 in]
              }
            }
            n152 = Enqueue Element(queue=w477, element=T8 {"GenericDAQ State"=enum."_WaitForDone/Idle", "Variant"=variant}, error in (no error)=w476) -> (error out=w486:errorcluster)  [unwired: 1 in, 2 out]
            n153 = Bundle By Name(cluster=w486, "source"=w478) -> (w479:errorcluster)
          }
          frame "GetStatus" {
            n154 = Unbundle By Name(w498) -> ("Handle"=w499:T11)
            n155 = call <instrlib>:"CsTool-QueryStatus.vi"("Handle Cluster"=w499) -> ("Status"=w497:i32)
            n156 = Bundle By Name(cluster=w498, "DAQ_Status"=w497) -> (w502:T1)
          }
          frame "_WaitForDone/Idle" {
            w517 = T9[] [enum."Close", enum."CloseAll", enum."Reset", enum."Quit", enum."Abort"] items=["Enumerate", "Open", "Close", "CloseAll", "Reset", "Quit", "==Settings==", "SetAcquisition_", "SetChannels_", "SetTrigger_", "SetAnalogTrigDetector_", "SetAll_AcquChTrig_", "fConfigurate", "fStart", "GetStatus", "_WaitForDone/Idle", "_GetData", "GetAcquisition", "GetChannels", "GetTrigger", "GetAll_AcquChTrig", "Abort", "==Messaging==", "_PushDataOut", "GetStat_", "GetConfig_", "==ModeSetup==", "SetSignalBuffer_", "SetMode_", "SetSecondaryDataRef._", "SetDynamicBuffer_", "==AnalogOut==", "GetChannelCount_AO", "fStart_AO", "SetChEnable_AO", "SetConfig_AO", "SetFuncData_AO", "SetOffset_AO_", "SetMasterNode_AO", "SetStates_AO", "SetSymetry_AO", "SetTriggerSource_AO", "==Trigger==", "ManualTrigger", "===Sync===", "LineStart", "LineEnd", "FrameStart", "FrameEnd", "EOL_PassThrough", "SOL_PassThrough"]
            # "to be considered \n\nwhat if system not configed??\nwhat status is that?"
            # "0 dne\n1 armed\n2 triggered\n3 transfering"
            n157 = Unbundle By Name(w522) -> ("Handle"=w512:T11)
            n158 = call <instrlib>:"CsTool-QueryStatus.vi"("Handle Cluster"=w512) -> ("Status"=w509:i32)
            n159 = Bundle By Name(cluster=w522, "DAQ_Status"=w509) -> (w521:T1)
            n160 = Preview Queue Element(queue=w531, timeout in ms (-1)=0, error in (no error)=w530) -> (queue out=w526:refnum<queue>, element=w519:T8, timed out?=w518:bool, error out=w525:errorcluster)
            n161 = Unbundle(w519) -> ("GenericDAQ State"=w514:T9)  [unwired: 1 out]
            n162 = Search 1D Array(1D array=w517, element=w514) -> (index of element=w516:i32)  [unwired: 1 in]
            n163 = Greater Or Equal To 0?(x=w516) -> (x >= 0?=w515:bool)
            n164 = Compound Arithmetic op=AND(w515, invert w518) -> (w513:bool)
            n165 = case shown="False" w513 {
              tunnel: w526 -> [w535 _]
              tunnel: w525 -> [w534 w552]
              tunnel: [w533 w552] -> w524
              tunnel: w509 -> [w532 _]
              frame False {
                n166 = case shown="2, Default" w532 {
                  tunnel: w535 -> [w536 w547 w551]
                  tunnel: w534 -> [w539 w546 w550]
                  tunnel: [w538 w545 w549] -> w533
                  frame 1 {
                    # "armed ??"
                    # "Typically, this is caused by config change\nduring acquisition. \nPush fConfig and fStart to continure  acuisition."
                    # "armed, not configed??"
                    n167 = for {
                      shift-right: [w542] -> w538
                      shift-left: w539 -> [w543]
                      tunnel: T8[] [{"GenericDAQ State"=enum."_WaitForDone/Idle", "Variant"=variant}] -> [w541] mode=indexing
                      tunnel: w536 -> [w540]
                      n168 = Enqueue Element(queue=w540, element=w541, error in (no error)=w543) -> (error out=w542:errorcluster)  [unwired: 1 in, 2 out]
                    }
                  }
                  frame 0 {
                    # "Done"
                    n169 = Enqueue Element(queue=w547, element=T8 {"GenericDAQ State"=enum."_GetData", "Variant"=variant}, error in (no error)=w546) -> (error out=w545:errorcluster)  [unwired: 1 in, 2 out]
                  }
                  frame 2, Default {
                    # "triggered"
                    # "triggered, others"
                    n170 = Enqueue Element(queue=w551, element=T8 {"GenericDAQ State"=enum."_WaitForDone/Idle", "Variant"=variant}, error in (no error)=w550) -> (error out=w549:errorcluster)  [unwired: 1 in, 2 out]
                  }
                }
              }
              frame True {
              }
            }
            n171 = Wait (ms)(milliseconds to wait=u32 0) -> ()  [unwired: 1 out]
          }
          frame "_GetData" {
            w562 = u32[] [0, 0, 0, 16]  # Mode Lookup Table
            n172 = Unbundle By Name(w587) -> ("Acquisition.Segment"=w558:u32, "Channels"=w574:T14, "Acquisition.Depth"=w571:dbl, "Acquisition.Start (0)"=w566:dbl)
            n173 = Unbundle By Name(w576) -> ("Mode(Gage)"=w559:T7)
            n174 = Unbundle By Name(w576) -> ("TrigCount"=w575:i32, "Option(SecondaryDataVI)"=w564:i32, "SecondaryDataVIRef"=w565:refnum<vi>, "Handle"=w561:T11, "cSegment"=w556:i32)
            n175 = Enqueue Element(queue=w581, element=T8 {"GenericDAQ State"=enum."_PushDataOut", "Variant"=variant}, error in (no error)=w579) -> (error out=w567:errorcluster)  [unwired: 1 in, 2 out]
            n176 = Array Size(array=w574) -> (size(s)=w568:i32)
            n177 = Index Array(array=w562, index=w559) -> (element=w553:u32)
            n178 = Decrement(x=w556) -> (x-1=w557:i32)
            n179 = Subtract(x=w558, y=w557) -> (x-y=w560:u32)
            n180 = for {
              N: w568 -> [_]
              tunnel: w586 -> [w650]
              tunnel: [w649] -> w578 mode=concatenating
              tunnel: w561 -> [w648]
              tunnel: w573 -> [w647]
              tunnel: w572 -> [w646]
              tunnel: w571 -> [w645]
              tunnel: [w644] -> w570 mode=concatenating
              tunnel: [w641] -> w569 mode=concatenating
              tunnel: w553 -> [w643]
              tunnel: w566 -> [w642]
              tunnel: [w641] -> _
              shift-right: [w640] -> w563
              shift-left: w567 -> [w640]
              tunnel: w560 -> [w638]
              i -> [w639]
              n181 = call <instrlib>:"GageTransfer-LowOverheadMod.vi"("Handle Cluster"=w648, "Start (0)"=w642, "Length (4096)"=w645, "Buffer in I32"=w650, "Buffer in I16"=w647, "Buffer in U8"=w646, "Channel (0)"=w639, "Mode (0)"=w643, "Segment (1)"=w638) -> ("Buffer Out I32"=w649:i32[], "Buffer Out I16"=w644:i16[], "Buffer Out U8"=w641:u8[])  [unwired: 1 in, 3 out]
            }
            n182 = Increment(x=w575) -> (x+1=w577:i32)
            n183 = Bundle By Name(cluster=w576, "TrigCount"=w577, "cSegment"=w557) -> (w555:T1)
            n184 = case shown="\"MultiRecord\"" w559 {
              tunnel: w584 -> [w600 w613 w634]
              tunnel: [w599 w613 w633] -> w583
              tunnel: [w598 w612 w629] -> w582
              tunnel: w561 -> [w597 w609 _]
              tunnel: w565 -> [w596 _ w632]
              tunnel: w564 -> [w595 _ w631]
              tunnel: w563 -> [w593 w611 w629]
              tunnel: w557 -> [_ w606 _]
              tunnel: w558 -> [_ w604 _]
              tunnel: w555 -> [w588 w608 w626]
              tunnel: [w588 w607 w626] -> w554
              frame "Continuous", Default {
                n185 = Not A Number/Path/Refnum?(number/path/refnum=w596) -> (NaN/Path/Refnum?=w591:bool)
                n186 = case shown="False" w591 {
                  tunnel: [w603 _] -> w592
                  tunnel: w596 -> [w602 _]
                  tunnel: w595 -> [w601 _]
                  frame False {
                    n187 = call-by-ref "?"(reference=w602, "Option"=w601) -> ("SecondaryData"=w603:dbl[])  [unwired: 11 in, 2 out]
                  }
                  frame True {
                  }
                }
                n188 = call <instrlib>:"CsTool-Capture.vi"("Handle Cluster"=w597) -> ("Error Code"=w590:i32)
                n189 = call <instrlib>:"CsTool-ErrorHandler.vi"("Error Code"=w590, "Handle Cluster"=w597) -> ("Error String"=w589:string)  [unwired: 1 in]
                n190 = Tick Count (ms)() -> (millisecond timer value=w594:u32)
                n191 = Bundle By Name(cluster=w600, "tickcount"=w594, "SecondaryData"=w592) -> (w599:T6)
                n192 = Bundle By Name(cluster=w593, "source"=w589) -> (w598:errorcluster)
              }
              frame "MultiRecord" {
                n193 = Increment(x=w606) -> (x+1=w605:i32)
                n194 = case shown="0" w606 {
                  tunnel: [w624 w625] -> w612
                  tunnel: w609 -> [w623 _]
                  tunnel: w611 -> [w622 w625]
                  frame 0 {
                    # "End of MultiRecord Transfer, start next"
                    n195 = call <instrlib>:"CsTool-Capture.vi"("Handle Cluster"=w623) -> ("Error Code"=w621:i32)
                    n196 = call <instrlib>:"CsTool-ErrorHandler.vi"("Error Code"=w621, "Handle Cluster"=w623) -> ("Error String"=w620:string)  [unwired: 1 in]
                    n197 = Bundle By Name(cluster=w622, "source"=w620) -> (w624:errorcluster)
                  }
                  frame Default {
                  }
                }
                n198 = Equal?(x=w604, y=w605) -> (x = y?=w610:bool)
                n199 = case shown="True" w610 {
                  tunnel: w609 -> [_ w619]
                  tunnel: w605 -> [_ w618]
                  tunnel: w608 -> [w614 w616]
                  tunnel: [w614 w615] -> w607
                  frame False {
                  }
                  frame True {
                    # "Get TS array at the first record"
                    n200 = call <instrlib>:"CsTool-TransferTimeStamp.vi"("Length (1)"=w618, "Handle Cluster"=w619) -> ("TS Time"=w617:dbl[])  [unwired: 1 in, 2 out]
                    n201 = Bundle By Name(cluster=w616, "TSArray"=w617) -> (w615:T1)
                  }
                }
              }
              frame "Normal" {
                n202 = Not A Number/Path/Refnum?(number/path/refnum=w632) -> (NaN/Path/Refnum?=w627:bool)
                n203 = case shown="False" w627 {
                  tunnel: [w637 _] -> w628
                  tunnel: w632 -> [w636 _]
                  tunnel: w631 -> [w635 _]
                  frame False {
                    n204 = call-by-ref "?"(reference=w636, "Option"=w635) -> ("SecondaryData"=w637:dbl[])  [unwired: 11 in, 2 out]
                  }
                  frame True {
                  }
                }
                n205 = Tick Count (ms)() -> (millisecond timer value=w630:u32)
                n206 = Bundle By Name(cluster=w634, "tickcount"=w630, "SecondaryData"=w628) -> (w633:T6)
              }
            }
          }
          frame "GetAcquisition" {
            # "Mode and Segment Count"
            n207 = Unbundle By Name(w670) -> ("Handle"=w654:T11)
            n208 = call <instrlib>:"CsTool-QueryAcquisitionParameters.vi"("Handle Cluster"=w654) -> ("Error Code"=w653:i32, "Trigger Holdoff"=w668:dbl, "Trigger Delay"=w667:dbl, "Output Handle Cluster"=w664:T19, "Sample Rate"=w666:dbl, "Clock Mode"=w663:enum16{"Internal", "External", "Reference"}, "Mode"=w656:string, "Trigger Timeout"=w660:dbl, "Segment Size"=w661:dbl, "Depth"=w662:dbl)  [unwired: 4 in, 1 out]
            n209 = call <instrlib>:"CsTool-ErrorHandler.vi"("Error Code"=w653, "Handle Cluster"=w654) -> ("Error String"=w651:string)  [unwired: 1 in]
            n210 = Bundle By Name(cluster=w674, "source"=w651) -> (w652:errorcluster)
            n211 = Bundle By Name(cluster=w670, "Handle"=w664) -> (w665:T1)
            n212 = Search 1D Array(1D array=string[] ["Single", "Dual", "Quad", "Octal"], element=w656) -> (index of element=w655:i32)  [unwired: 1 in]
            n213 = Bundle By Name(cluster=w671, "Acquisition.Sample Rate"=w666, "Acquisition.Mode"=w655, "Acquisition.Depth"=w662, "Acquisition.Segment Size"=w661, "Acquisition.Trigger Timeout"=w660, "Acquisition.Trigger Holdoff"=w668, "Acquisition.Trigger Delay"=w667, "Acquisition.Clock mode"=w663) -> (w669:T3)
          }
          frame "GetChannels" {
            n214 = Unbundle By Name(w684) -> ("Handle"=w686:T11)
            n215 = Unbundle By Name(w683) -> ("Channels"=w682:T14)
            n216 = for {
              tunnel: w686 -> [w692]
              tunnel: w682 -> [w704] mode=indexing
              tunnel: [w697] -> w681 mode=indexing
              tunnel: [w691] -> w677 mode=indexing
              i -> [w705]
              n217 = call <instrlib>:"CsTool-QueryChannelParameters.vi"("Handle Cluster"=w692, "Channel"=w705) -> ("Filter"=w698:u32, "Coupling"=w695:string, "Differential Input"=w703:bool, "Direct-to-ADC"=w699:bool, "Range (mV)"=w702:u32, "Impedance"=w701:u32, "DC Offset (mV)"=w700:u32, "Error Code"=w693:i32)
              n218 = call <instrlib>:"CsTool-ErrorHandler.vi"("Error Code"=w693, "Handle Cluster"=w692) -> ("Error String"=w691:string)  [unwired: 1 in]
              n219 = Search 1D Array(1D array=string[] ["DC", "AC"], element=w695) -> (index of element=w694:i32)  [unwired: 1 in]
              n220 = Bundle By Name(cluster=w704, "Differential Input"=w703, "Range"=w702, "Impedance"=w701, "DC Offset"=w700, "Direct-to-ADC"=w699, "Coupling"=w694, "Filter"=w698) -> (w697:T20)
            }
            n221 = Concatenate Strings(w677) -> (w676:string)
            n222 = Bundle By Name(cluster=w683, "Channels"=w681) -> (w685:T3)
            n223 = Bundle By Name(cluster=w689, "source"=w676) -> (w678:errorcluster)
          }
          frame "GetTrigger" {
            n224 = Unbundle By Name(w726) -> ("Handle"=w708:T11)
            n225 = call <instrlib>:"CsTool-QueryTriggerParameters.vi"("Handle Cluster"=w708, "Trigger"=u32 0) -> ("External Impedance"=w712:string, "External Range (mV)"=w724:u32, "External Coupling"=w715:string, "Error Code"=w709:i32, "Source"=w723:i32, "Slope"=w718:string, "Level"=w722:i32, "External Trigger"=w721:bool, "Disable Trigger"=w720:bool)  [unwired: 9 in]
            n226 = call <instrlib>:"CsTool-ErrorHandler.vi"("Error Code"=w709, "Handle Cluster"=w708) -> ("Error String"=w706:string)  [unwired: 1 in]
            n227 = Search 1D Array(1D array=string[] ["rising", "falling"], element=w718) -> (index of element=w717:i32)  [unwired: 1 in]
            n228 = Search 1D Array(1D array=string[] ["dc", "ac"], element=w715) -> (index of element=w714:i32)  [unwired: 1 in]
            n229 = Search 1D Array(1D array=string[] ["50 Ohm", "HiZ"], element=w712) -> (index of element=w711:i32)  [unwired: 1 in]
            n230 = Bundle By Name(cluster=w732, "source"=w706) -> (w707:errorcluster)
            n231 = Bundle By Name(cluster=w731, "Trigger.External Range"=w724, "Trigger.Source"=w723, "Trigger.Slope"=w717, "Trigger.Level"=w722, "Trigger.External"=w721, "Trigger.Disable"=w720, "Trigger.External Coupling"=w714, "Trigger.External Impedance"=w711) -> (w725:T3)
          }
          frame "GetAll_AcquChTrig" {
            n232 = for "Has to be at the \nopposite end, otherwise\nrace condition" {
              tunnel: w737 -> [w748]
              shift-right: [w747] -> w735
              shift-left: w736 -> [w746]
              tunnel: T8[] [{"GenericDAQ State"=enum."GetAcquisition", "Variant"=variant}, {"GenericDAQ State"=enum."GetChannels", "Variant"=variant}, {"GenericDAQ State"=enum."GetTrigger", "Variant"=variant}] -> [w745] mode=indexing
              n233 = Enqueue Element At Opposite End(queue=w748, element=w745, error in (no error)=w746) -> (error out=w747:errorcluster)  [unwired: 1 in, 2 out]
            }
          }
          frame "Abort" {
            n234 = call <instrlib>:"CleanupDAQTasks.vi"("error in (no error)"=w750, "Queue in"=w751) -> ("error out"=w749:errorcluster)  [unwired: 8 in, 1 out]
            n235 = Unbundle By Name(w752) -> ("Handle"=w753:T11)
            n236 = call <instrlib>:"CsTool-AbortCapture.vi"("Handle Cluster"=w753) -> ()  [unwired: 1 out]
          }
          frame "==Messaging==" {
            # "Invalid Frame"
            n237 = xnode "Error Ring"() -> ("error out"=w762:errorcluster)
          }
          frame "_PushDataOut" {
            n238 = Unbundle By Name(w782) -> ("Mode(Gage)"=w799:T7)
            n239 = Unbundle By Name(w791) -> ("Channels"=w790:T14, "Acquisition.Segment"=w780:u32)
            n240 = Unbundle By Name(w782) -> ("TSArray"=w774:dbl[], "cSegment"=w779:i32, "Handle.Resolution"=w783:i32, "Handle.Sample size"=w795:u32, "Handle.Offset"=w792:i32)
            n241 = case "ADC counts to Voltage conversion (for compatibility)" shown="4" w795 {
              tunnel: w785 -> [w804 w817 w834]
              tunnel: [w807 w822 w837] -> w793
              tunnel: w787 -> [w803 w818 w833]
              tunnel: w789 -> [w802 w819 w832]
              tunnel: w792 -> [w806 w821 w836]
              tunnel: w790 -> [w805 w820 w835]
              tunnel: [w802 w819 w832] -> w788
              tunnel: [w803 w818 w833] -> w786
              tunnel: [w804 w817 w834] -> w784
              tunnel: w783 -> [w801 w816 w831]
              frame 4 {
                n242 = for {
                  tunnel: w802 -> [w815]
                  tunnel: [w809] -> w807 mode=concatenating
                  tunnel: w801 -> [w814]
                  tunnel: w806 -> [w813]
                  tunnel: w805 -> [w812] mode=indexing
                  n243 = Unbundle By Name(w812) -> ("DC Offset"=w811:i32, "Range"=w810:u32)
                  n244 = To Single Precision Float(number=w815) -> (single precision float=w808:sgl[])
                  n245 = call <instrlib>:"ConvertTo_DBL.vi"("Input Range (mV)"=w810, "DC Offset (mV)"=w811, "Offset"=w813, "Resolution"=w814, "Interger Signal"=w808) -> ("Data (V)"=w809:sgl[])  [unwired: 6 in]
                }
              }
              frame 2 {
                n246 = for {
                  tunnel: w818 -> [w830]
                  tunnel: [w824] -> w822 mode=concatenating
                  tunnel: w816 -> [w829]
                  tunnel: w821 -> [w828]
                  tunnel: w820 -> [w827] mode=indexing
                  n247 = Unbundle By Name(w827) -> ("DC Offset"=w826:i32, "Range"=w825:u32)
                  n248 = To Single Precision Float(number=w830) -> (single precision float=w823:sgl[])
                  n249 = call <instrlib>:"ConvertTo_DBL.vi"("Input Range (mV)"=w825, "DC Offset (mV)"=w826, "Offset"=w828, "Resolution"=w829, "Interger Signal"=w823) -> ("Data (V)"=w824:sgl[])  [unwired: 6 in]
                }
              }
              frame 1, Default {
                n250 = for {
                  tunnel: w834 -> [w845]
                  tunnel: [w838] -> w837 mode=concatenating
                  tunnel: w831 -> [w844]
                  tunnel: w836 -> [w843]
                  tunnel: w835 -> [w842] mode=indexing
                  n251 = Unbundle By Name(w842) -> ("DC Offset"=w841:i32, "Range"=w840:u32)
                  n252 = To Single Precision Float(number=w845) -> (single precision float=w839:sgl[])
                  n253 = call <instrlib>:"ConvertTo_DBL.vi"("Input Range (mV)"=w840, "DC Offset (mV)"=w841, "Offset"=w843, "Resolution"=w844, "Interger Signal"=w839) -> ("Data (V)"=w838:sgl[])  [unwired: 6 in]
                }
              }
            }
            n254 = case shown="\"MultiRecord\"" w799 {
              tunnel: w798 -> [w847 w854 w874]
              tunnel: [w847 w853 w873] -> w797
              tunnel: w796 -> [_ w852 w872]
              tunnel: w782 -> [w846 w850 w871]
              tunnel: [w846 w849 w870] -> w781
              tunnel: w780 -> [_ w848 w861]
              tunnel: w779 -> [_ _ w860]
              tunnel: [_ _ TRUE] -> w777
              tunnel: w774 -> [_ _ w859]
              tunnel: [_ _ w855] -> w773
              frame "Normal" {
              }
              frame "Continuous", Default {
                # "In continuous single trigger  mode, \nre-arming is done in \"_GetData\"\n\nNormal mode => no need to re-arming  daq"
                n255 = Enqueue Element(queue=w852, element=T8 {"GenericDAQ State"=enum."_WaitForDone/Idle", "Variant"=variant}, error in (no error)=w854) -> (error out=w853:errorcluster)  [unwired: 1 in, 2 out]
                n256 = Bundle By Name(cluster=w850, "cSegment"=w848) -> (w849:T1)
              }
              frame "MultiRecord" {
                # "3 functions:\n1. retrival of timestamp\n2. reset cSegment counter\n3. decide continue transfer or wait for next round"
                n257 = Subtract(x=w861, y=w860) -> (x-y=w862:u32)
                n258 = Equal To 0?(x=w860) -> (x = 0?=w868:bool)
                n259 = Decrement "Get Index"(x=w862) -> (x-1=w863:u32)
                n260 = Index Array(array=w859, index=w863) -> (element=w858:dbl)
                n261 = Select(t=w861, s=w868, f=w860) -> (s? t:f=w869:u32)
                n262 = Select(t=T8 {"GenericDAQ State"=enum."_WaitForDone/Idle", "Variant"=variant} ("element"), s=w868, f=T8 {"GenericDAQ State"=enum."_GetData", "Variant"=variant} ("element")) -> (s? t:f=w865:T8)
                n263 = Multiply(x=w858, y=1000.0) -> (x*y=w857:dbl)
                n264 = Bundle By Name(cluster=w871, "cSegment"=w869) -> (w870:T1)
                n265 = Enqueue Element(queue=w872, element=w865, error in (no error)=w874) -> (error out=w873:errorcluster)  [unwired: 1 in, 2 out]
                n266 = To Unsigned Long Integer(number=w857) -> (unsigned 32bit integer=w855:u32)
              }
            }
            n267 = Unbundle By Name(w775) -> ("tickcount"=w776:u32)
            n268 = Select(t=w773, s=w777, f=w776) -> (s? t:f=w778:u32)
            n269 = Bundle By Name(cluster=w775, "Signal"=w793, "tickcount"=w778) -> (w794:T6)
            n270 = Enqueue Element "Send/Push Data Out"(queue=w800, element=w794) -> ()  [unwired: 2 in, 3 out]
          }
          frame "GetStat_" {
            n271 = Variant To Data(error in=w881, type=refnum<queue> refnum ("queue out"), Variant=w882) -> (data=w884:refnum<queue>, error out=w883:errorcluster)
            n272 = Enqueue Element "Send Core Stat"(queue=w884, element=w876, error in (no error)=w883) -> (error out=w880:errorcluster)  [unwired: 1 in, 2 out]
          }
          frame "GetConfig_" {
            # "solution:\n\n1 call vi ref, vi send out typed command. => possible, idea, time consuming \n\n2 make this frame specific, bad. \n\n3 user event call and wait, then send typed command.  possible, fast?"
            n273 = Variant To Data(type=refnum<queue> refnum ("queue out"), Variant=w896) -> (data=w895:refnum<queue>, error out=w894:errorcluster)  [unwired: 1 in]
            n274 = case shown="No Error" w894 {
              selector: w894 -> [_ w905]
              tunnel: w895 -> [w904 _]
              tunnel: w893 -> [w901 _]
              tunnel: [w903 w905] -> w892
              tunnel: w891 -> [w902 _]
              frame No Error {
                # "short term solution, need refine\nget real result from device"
                n275 = Enqueue Element(queue=w904, element=w901, error in (no error)=w902) -> (error out=w903:errorcluster)  [unwired: 1 in, 2 out]
              }
              frame Error {
              }
            }
          }
          frame "==ModeSetup==" {
            # "Invalid Frame"
            n276 = xnode "Error Ring"() -> ("error out"=w908:errorcluster)
          }
          frame "SetSignalBuffer_" {
            n277 = Variant To Data(type=w926, Variant=w928) -> (data=w925:refnum<queue>, error out=w922:errorcluster)  [unwired: 1 in]
            n278 = Select(t=w926, s=w922, f=w925) -> (s? t:f=w927:refnum<queue>)
            n279 = xnode "Error Ring"() -> ("error out"=w921:errorcluster)
            n280 = Select(t=w921, s=w922, f=w923) -> (s? t:f=w924:errorcluster)
          }
          frame "SetMode_" {
            n281 = Unbundle By Name(w947) -> ("Mode(Gage)"=w945:T7, "Handle"=w938:T11)
            n282 = Variant To Data(error in=w942, type=w945, Variant=w946) -> (data=w944:T7, error out=w943:errorcluster)
            n283 = Select(t=w945, s=w943, f=w944) -> (s? t:f=w939:T7)
            n284 = Bundle By Name(cluster=w947, "Mode(Gage)"=w939) -> (w948:T1)
            n285 = case shown="\"MultiRecord\"" w939 {
              tunnel: w938 -> [w953 _]
              frame "MultiRecord" {
                # "for multirecord  and hwaverage"
                n286 = call <instrlib>:"CsTool-ConfigureTimeStamp.vi"("Handle Cluster"=w953) -> ()  [unwired: 2 in, 1 out]
              }
              frame Default {
              }
            }
          }
          frame "SetSecondaryDataRef._" {
            n287 = Variant To Data(type=T10 {"SecondaryDataVIRef."=refnum, "Option"=0} ("SecondaryDataParams."), Variant=w958) -> (data=w956:T10, error out=w957:errorcluster)  [unwired: 1 in]
            n288 = case shown="No Error" w957 {
              tunnel: w955 -> [w980 w984]
              tunnel: [w979 w984] -> w960
              tunnel: w956 -> [w975 _]
              tunnel: w955 -> [w972 _]
              tunnel: [w967 w983] -> w954
              frame No Error {
                n289 = Unbundle By Name(w972) -> ("SecondaryDataVIRef"=w970:refnum<vi>)
                n290 = Unbundle By Name(w975) -> ("SecondaryDataVIRef."=w974:refnum<vi>, "Option"=w973:i32)
                n291 = Not A Number/Path/Refnum?(number/path/refnum=w970) -> (NaN/Path/Refnum?=w971:bool)
                n292 = case shown="False" w971 {
                  tunnel: w970 -> [w982 _]
                  tunnel: [w981 _] -> w969
                  frame False {
                    n293 = Close Reference(reference=w982) -> (error out=w981:errorcluster)  [unwired: 1 in]
                  }
                  frame True {
                  }
                }
                n294 = property class="VI Interface Type 0"(reference=w974, error in=w969) -> (reference out=w977:refnum<vi>, error out=w968:errorcluster, "Path"=w978:path)
                n295 = Open VI Reference(type specifier VI Refnum (for type only)=w977, vi path=w978, error in (no error)=w968) -> (vi reference=w976:refnum<vi>, error out=w967:errorcluster)  [unwired: 3 in]
                n296 = Bundle By Name(cluster=w980, "SecondaryDataVIRef"=w976, "Option(SecondaryDataVI)"=w973) -> (w979:T1)
              }
              frame Error {
                n297 = xnode "Error Ring"() -> ("error out"=w983:errorcluster)
              }
            }
          }
          frame "===Sync===" {
          }
          frame "LineStart", "SOL_PassThrough" {
            n298 = Enqueue Element(queue=w998, element=T6 {"tickcount"=0, "Signal"=[], "SecondaryData"=[], "Flag"=enum."LineStart", "Segment#"=1}) -> ()  [unwired: 2 in, 3 out]
          }
          frame "LineEnd", "EOL_PassThrough" {
            n299 = Enqueue Element(queue=w1007, element=T6 {"tickcount"=0, "Signal"=[], "SecondaryData"=[], "Flag"=enum."LineEnd", "Segment#"=1}) -> ()  [unwired: 2 in, 3 out]
          }
        }
      }
      frame Error {
        n300 = xnode "Error Ring"() -> ("error out"=w1018:errorcluster)
      }
    }
    n301 = call <userlib>:"ErrorLog.vi"("error in (no error)"=w51) -> ("error out"=w50:errorcluster)  [unwired: 10 in]
    "Core#" <- w52
  }
  "error out" <- w16
  n302 = while {
    tunnel: w23 -> [w1037]
    tunnel: w6 -> [w1036]
    tunnel: w21 -> [w1034]
    tunnel: w11 -> [w1033]
    tunnel: [w1032] -> w9
    tunnel: [w1031] -> _
    tunnel: [w1030] -> _
    stop <- w1030 stop-if-true
    w1035 = 500  # Should not be -1, or do not quit as subVI
    n303 = event shown="[13] \"Open\": Value Change" {
      selector: _ -> [_ _ _ _ _ _ _ _ _ _ _ _ _ _ _ _]
      dyn-events: _ -> [_ _ _ _ _ _ _ _ _ _ _ _ _ _ _ _]
      timeout: w1035 -> [w1039 _ _ _ _ _ _ _ _ _ _ _ _ _ _ _]
      tunnel: w1037 -> [w1048 w1064 w1068 w1072 w1077 w1079 w1087 w1091 w1093 w1095 w1097 w1099 w1101 w1103 w1105 w1107]
      tunnel: w1036 -> [_ _ _ _ w1074 _ _ _ _ _ _ _ _ _ _ _]
      tunnel: w1034 -> [w1047 _ _ _ _ _ _ _ _ _ _ _ _ _ _ _]
      tunnel: [_ _ _ _ _ _ TRUE _ _ _ _ _ _ _ _ _] -> w1031
      tunnel: [w1046 _ _ _ _ _ errorcluster {"status"=FALSE, "code"=0, "source"=""} ("error constant") _ _ _ _ _ _ _ _ _] -> w1032
      event Timeout {
        n304 = event-data() -> ()  [unwired: 1 in, 1 out]
        n305 = Bundle By Name(cluster=T8 {"GenericDAQ State"=enum."GetStat_", "Variant"=variant} ("element"), "Variant"=w1047) -> (w1044:T8)
        n306 = Enqueue Element At Opposite End "To get LiveStat,\nIt has to be opposite end"(queue=w1048, element=w1044) -> (error out=w1043:errorcluster)  [unwired: 2 in, 2 out]
        n307 = Dequeue Element(queue=w1047, timeout in ms (-1)=100, error in (no error)=w1043) -> (element=w1042:T1, timed out?=w1040:bool, error out=w1046:errorcluster)  [unwired: 1 out]
        n308 = case shown="False" w1040 {
          tunnel: w1042 -> [w1057 w1060]
          tunnel: [w1056 w1059] -> w1041
          tunnel: w1039 -> [w1052 _]
          frame False {
            n309 = Unbundle By Name(w1057) -> ("TrigCount"=w1055:i32)
            n310 = feedback-in #1(w1055) -> ()
            n311 = feedback #1(0 ("TrigCount")) -> (w1054:i32)
            n312 = Subtract(x=w1055, y=w1054) -> (x-y=w1053:i32)
            n313 = Compound Arithmetic op=MULTIPLY(w1053, invert w1052, 1000.0 ("value")) -> (w1050:dbl)
            n314 = Bundle By Name(cluster=w1057, "TrigRate(Hz)"=w1050) -> (w1056:T1)
          }
          frame True {
            n315 = Bundle By Name(cluster=w1060, "Model"="timeout !") -> (w1059:T1)
          }
        }
        "LiveStat" <- w1041
      }
      event Value Change {
        n316 = event-data() -> ("NewVal"=w1061:T12)  [unwired: 1 in]
        n317 = Bundle By Name(cluster=T8 {"GenericDAQ State"=enum."SetAcquisition_", "Variant"=variant} ("element"), "Variant"=w1061) -> (w1062:T8)
        n318 = Enqueue Element(queue=w1064, element=w1062) -> ()  [unwired: 2 in, 3 out]
      }
      event Value Change {
        n319 = event-data() -> ("NewVal"=w1065:T14)  [unwired: 1 in]
        n320 = Bundle By Name(cluster=T8 {"GenericDAQ State"=enum."SetChannels_", "Variant"=variant} ("element"), "Variant"=w1065) -> (w1066:T8)
        n321 = Enqueue Element(queue=w1068, element=w1066) -> ()  [unwired: 2 in, 3 out]
      }
      event Value Change {
        n322 = event-data() -> ("NewVal"=w1069:T16)  [unwired: 1 in]
        n323 = Bundle By Name(cluster=T8 {"GenericDAQ State"=enum."SetTrigger_", "Variant"=variant} ("element"), "Variant"=w1069) -> (w1070:T8)
        n324 = Enqueue Element(queue=w1072, element=w1070) -> ()  [unwired: 2 in, 3 out]
      }
      event "ConfigAll": Value Change {
        n325 = event-data() -> ()  [unwired: 1 in, 1 out]
        n326 = property class="Clust (strict)"(reference=w1074) -> ("Value"=w1073:T21)  [unwired: 1 in, 2 out]
        n327 = Bundle By Name(cluster=T8 {"GenericDAQ State"=enum."SetAll_AcquChTrig_", "Variant"=variant} ("element"), "Variant"=w1073) -> (w1075:T8)
        n328 = Enqueue Element(queue=w1077, element=w1075) -> ()  [unwired: 2 in, 3 out]
      }
      event "Get_ConfigAll": Value Change {
        n329 = event-data() -> ()  [unwired: 1 in, 1 out]
        n330 = for {
          tunnel: w1079 -> [w1083]
          shift-right: [w1082] -> _
          shift-left: _ -> [w1081]
          tunnel: T8[] [{"GenericDAQ State"=enum."GetAcquisition", "Variant"=variant}, {"GenericDAQ State"=enum."GetChannels", "Variant"=variant}, {"GenericDAQ State"=enum."GetTrigger", "Variant"=variant}] -> [w1080] mode=indexing
          n331 = Enqueue Element(queue=w1083, element=w1080, error in (no error)=w1081) -> (error out=w1082:errorcluster)  [unwired: 1 in, 2 out]
        }
      }
      event "Quit": Value Change {
        n332 = event-data() -> ()  [unwired: 1 in, 1 out]
        n333 = Enqueue Element(queue=w1087, element=T8 {"GenericDAQ State"=enum."Quit", "Variant"=variant}) -> ()  [unwired: 2 in, 3 out]
      }
      event Value Change {
        n334 = event-data() -> ("NewVal"=w1088:T7)  [unwired: 1 in]
        n335 = Bundle By Name(cluster=T8 {"GenericDAQ State"=enum."SetMode_", "Variant"=variant} ("element"), "Variant"=w1088) -> (w1089:T8)
        n336 = Enqueue Element(queue=w1091, element=w1089) -> ()  [unwired: 2 in, 3 out]
      }
      event "fConfig": Value Change {
        n337 = event-data() -> ()  [unwired: 1 in, 1 out]
        n338 = Enqueue Element(queue=w1093, element=T8 {"GenericDAQ State"=enum."fConfigurate", "Variant"=variant}) -> ()  [unwired: 2 in, 3 out]
      }
      event "Start": Value Change {
        n339 = event-data() -> ()  [unwired: 1 in, 1 out]
        n340 = Enqueue Element(queue=w1095, element=T8 {"GenericDAQ State"=enum."fStart", "Variant"=variant}) -> ()  [unwired: 2 in, 3 out]
      }
      event "Reset": Value Change {
        n341 = event-data() -> ()  [unwired: 1 in, 1 out]
        n342 = Enqueue Element(queue=w1097, element=T8 {"GenericDAQ State"=enum."Quit", "Variant"=variant}) -> ()  [unwired: 2 in, 3 out]
      }
      event "CloseAll": Value Change {
        n343 = event-data() -> ()  [unwired: 1 in, 1 out]
        n344 = Enqueue Element(queue=w1099, element=T8 {"GenericDAQ State"=enum."CloseAll", "Variant"=variant}) -> ()  [unwired: 2 in, 3 out]
      }
      event "Close": Value Change {
        n345 = event-data() -> ()  [unwired: 1 in, 1 out]
        n346 = Enqueue Element(queue=w1101, element=T8 {"GenericDAQ State"=enum."Close", "Variant"=variant}) -> ()  [unwired: 2 in, 3 out]
      }
      event "Open": Value Change {
        n347 = event-data() -> ()  [unwired: 1 in, 1 out]
        n348 = Enqueue Element(queue=w1103, element=T8 {"GenericDAQ State"=enum."Open", "Variant"=variant}) -> ()  [unwired: 2 in, 3 out]
      }
      event "Enumerate": Value Change {
        n349 = event-data() -> ()  [unwired: 1 in, 1 out]
        n350 = Enqueue Element(queue=w1105, element=T8 {"GenericDAQ State"=enum."Enumerate", "Variant"=variant}) -> ()  [unwired: 2 in, 3 out]
      }
      event "StartAll": Value Change {
        n351 = event-data() -> ()  [unwired: 1 in, 1 out]
        n352 = property on="Gage_Config" class="Clust (strict)"() -> ("Value"=w1106:T21)  [unwired: 2 in, 2 out]
        n353 = Bundle By Name(cluster=T8 {"GenericDAQ State"=enum."SetAll_AcquChTrig_", "Variant"=variant} ("element"), "Variant"=w1106) -> (w1111:T8)
        n354 = Build Array(T8 {"GenericDAQ State"=enum."Enumerate", "Variant"=variant} ("element"), T8 {"GenericDAQ State"=enum."Open", "Variant"=variant} ("element"), w1111, T8 {"GenericDAQ State"=enum."fConfigurate", "Variant"=variant} ("element"), T8 {"GenericDAQ State"=enum."fStart", "Variant"=variant} ("element")) -> (w1114:T8[])
        n355 = for {
          shift-right: [w1118] -> _
          shift-left: w1107 -> [w1119]
          tunnel: w1114 -> [w1117] mode=indexing
          shift-right: [w1116] -> _
          shift-left: _ -> [w1115]
          n356 = Enqueue Element(queue=w1119, element=w1117, error in (no error)=w1115) -> (queue out=w1118:refnum<queue>, error out=w1116:errorcluster)  [unwired: 1 in, 1 out]
        }
      }
    }
    n357 = Or(x=w1031, y=w1033) -> (x .or. y?=w1030:bool)
  }
  n358 = Release Queue(queue=w18, error in (no error)=w16) -> (error out=w22:errorcluster)  [unwired: 1 in, 2 out]
  n359 = Release Queue(queue=w23, error in (no error)=w22) -> (error out=w20:errorcluster)  [unwired: 1 in, 2 out]
  n360 = Merge Errors(w9, w20) -> (w10:errorcluster)
  n361 = Release Queue(queue=w21, error in (no error)=w10) -> (error out=w15:errorcluster)  [unwired: 1 in, 2 out]
  n362 = call <vilib>:"General Error Handler.vi"("type of dialog (OK msg:1)"=w14, "error in (no error)"=w15, "[exception action] (none:0)"=w13, "[exception code]"=w12) -> ()  [unwired: 7 in, 5 out]
